vi "DSF.Engine.BuilderManager.Pool.Obtain Builder.vi"(8 "error in (no error)":errorcluster, 9 "timeout in ms (250)":i32=250 format="%d ms", 11 "Builder Manager in":refnum<class "DSF.Engine.BuilderManager.lvclass">) -> (0 "error out":errorcluster, 2 "Builder":refnum<class "DSF.Engine.Builder.lvclass">, 3 "Builder Manager out":refnum<class "DSF.Engine.BuilderManager.lvclass">)   [LabVIEW 2017, in "DSF.Engine.lvlib" / "DSF.Engine.BuilderManager.lvclass"]
uses:
  DSF.Engine.BuilderManager.lvclass
  Builder/DSF.Engine.Builder.lvclass
  DSF.Engine.BuilderManager.lvclass/DSF.Engine.BuilderManager.ctl
  DSF.Engine.BuilderManager.Get Builders.vi
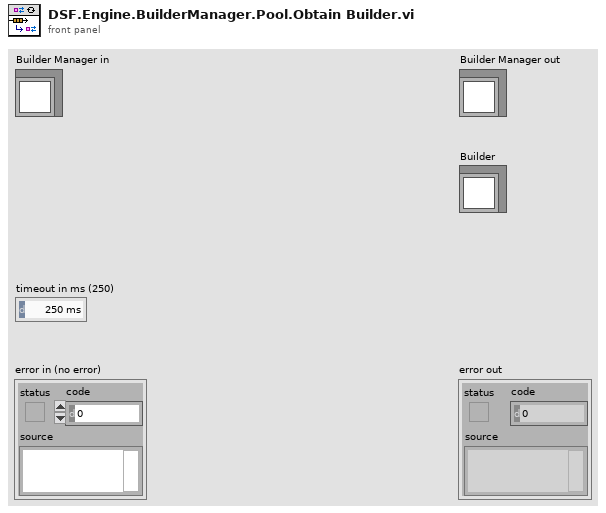
[diagram p1: front panel]
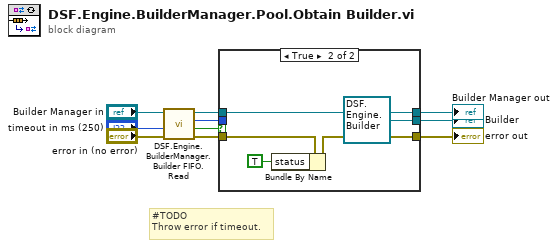
[diagram p0: block diagram]
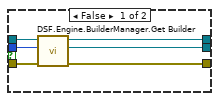
[diagram p2: hidden frame]
diagram:
  # "#TODO\nThrow error if timeout."
  n1 = call "DSF.Engine.BuilderManager.Builder FIFO.Read.vi"("error in (no error)"="error in (no error)", "timeout in ms (0)"="timeout in ms (250)", "Builder Manager in"="Builder Manager in") -> ("error out"=w7:errorcluster, "timed out?"=w6:bool, "Builder ID"=w5:i32, "Builder Manager out"=w4:refnum<class "DSF.Engine.BuilderManager.lvclass">)  [unwired: 5 in]
  n2 = case shown="True" w6 {
    tunnel: w7 -> [w12 w17]
    tunnel: w5 -> [w14 _]
    tunnel: w4 -> [w15 w20]
    tunnel: [w13 w20] -> w3
    tunnel: [w12 w16] -> w2
    tunnel: [w11 refnum<class "DSF.Engine.Builder.lvclass"> refnum ("Builder")] -> w1
    frame False {
      n3 = call "DSF.Engine.BuilderManager.Get Builder.vi"("ID"=w14, "Builder Manager in"=w15) -> ("Builder"=w11:refnum<class "DSF.Engine.Builder.lvclass">, "Builder Manager out"=w13:refnum<class "DSF.Engine.BuilderManager.lvclass">)  [unwired: 8 in]
    }
    frame True {
      n4 = Bundle By Name(cluster=w17, "status"=TRUE) -> (w16:errorcluster)
    }
  }
  "error out" <- w2
  "Builder Manager out" <- w3
  "Builder" <- w1
